vi "Display n or dt.vi"(8 "error in (no error)":errorcluster, 9 "Display n?":bool, 11 "Input Waveforms":waveform(dbl)[](array[waveform])) -> (0 "error out":errorcluster, 3 "Output Waveforms":waveform(dbl)[](array[waveform]))   [LabVIEW 2016, in "Instrument.Lockin.lvclass"]
uses:
  Instrument.Lockin.lvclass
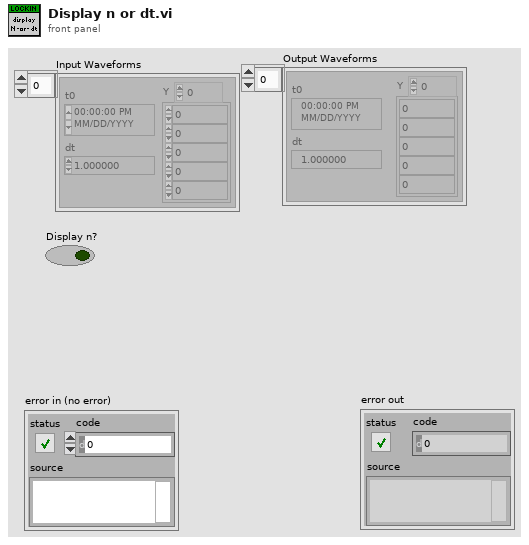
[diagram p1: front panel]
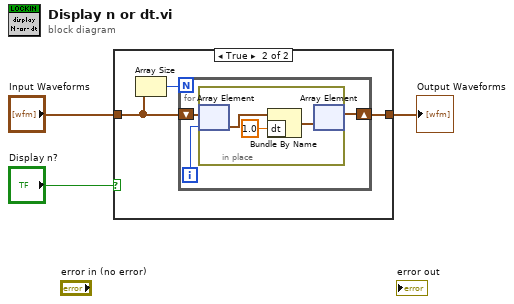
[diagram p0: block diagram]
diagram:
  n1 = case shown="True" "Display n?" {
    tunnel: [w4 w7] -> w3
    tunnel: "Input Waveforms" -> [w4 w5]
    frame False {
    }
    frame True {
      n2 = Array Size(array=w5) -> (size(s)=w6:i32)
      n3 = for {
        N: w6 -> [_]
        shift-right: [w8] -> w7
        shift-left: w5 -> [w9]
        i -> [w10]
        n4 = in-place {
          n5 = in-place-array #1(w9, w10) -> (w11:waveform(dbl))
          n6 = Bundle By Name(cluster=w11, "dt"=1.0) -> (w12:waveform(dbl))
          n7 = in-place-array #1(w12) -> (w8:waveform(dbl)[])  [unwired: 1 out]
        }
      }
    }
  }
  "Output Waveforms" <- w3
